vi "xy_graph_copy_format.vi"(6 "xy_scales_to_copy":i32=1, 8 "error in (no error)":errorcluster, 10 "destination":refnum<vi>, 11 "source":refnum<vi>) -> (0 "error out":errorcluster)   [LabVIEW 2015, in "lv-graph.lvlib"]
uses:
  lv-graph.lvlib
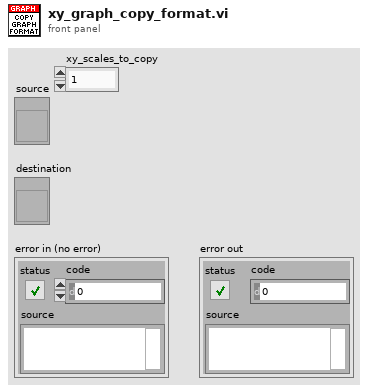
[diagram p1: front panel]
types:
  T1 = typedef "LVRangeTypeDef.ctl" = cluster{"Minimum":dbl, "Maximum":dbl, "Increment":dbl, "Minor Increment":dbl, "Start":dbl}
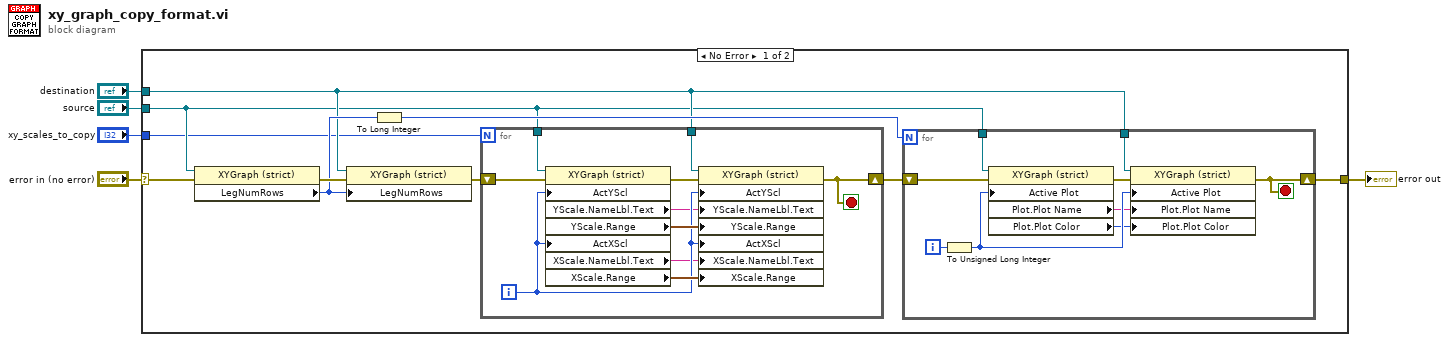
[diagram p0: block diagram]
diagram:
  n1 = case shown="No Error" "error in (no error)" {
    selector: "error in (no error)" -> [w7 w35]
    tunnel: [w12 w35] -> w5
    tunnel: "destination" -> [w9 _]
    tunnel: "source" -> [w8 _]
    tunnel: "xy_scales_to_copy" -> [w6 _]
    frame No Error {
      n2 = property class="XYGraph (strict)"(reference=w8, error in=w7) -> (error out=w15:errorcluster, "LegNumRows"=w14:u32)  [unwired: 1 out]
      n3 = property on="Property Node" class="XYGraph (strict)"(reference=w9, error in=w15, "LegNumRows"=w14) -> (error out=w11:errorcluster)  [unwired: 1 out]
      n4 = To Long Integer(number=w14) -> (32bit integer=w13:i32)
      n5 = for {
        N: w6 -> [_]
        shift-right: [w22] -> w10
        shift-left: w11 -> [w23]
        tunnel: w8 -> [w21]
        tunnel: w9 -> [w20]
        i -> [w18]
        stop <- w22 stop-if-true
        n6 = property on="Property Node" class="XYGraph (strict)"(reference=w21, error in=w23, "ActYScl"=w18, "ActXScl"=w18) -> (error out=w25:errorcluster, "YScale.NameLbl.Text"=w16:string, "YScale.Range"=w24:T1, "XScale.NameLbl.Text"=w17:string, "XScale.Range"=w19:T1)  [unwired: 1 out]
        n7 = property on="Property Node" class="XYGraph (strict)"(reference=w20, error in=w25, "ActYScl"=w18, "YScale.NameLbl.Text"=w16, "YScale.Range"=w24, "ActXScl"=w18, "XScale.NameLbl.Text"=w17, "XScale.Range"=w19) -> (error out=w22:errorcluster)  [unwired: 1 out]
      }
      n8 = for {
        N: w13 -> [_]
        shift-right: [w28] -> w12
        shift-left: w10 -> [w33]
        tunnel: w9 -> [w27]
        tunnel: w8 -> [w26]
        i -> [w32]
        stop <- w28 stop-if-true
        n9 = To Unsigned Long Integer(number=w32) -> (unsigned 32bit integer=w34:u32)
        n10 = property class="XYGraph (strict)"(reference=w26, error in=w33, "Active Plot"=w34) -> (error out=w31:errorcluster, "Plot.Plot Name"=w30:string, "Plot.Plot Color"=w29:u32)  [unwired: 1 out]
        n11 = property on="Property Node" class="XYGraph (strict)"(reference=w27, error in=w31, "Active Plot"=w34, "Plot.Plot Name"=w30, "Plot.Plot Color"=w29) -> (error out=w28:errorcluster)  [unwired: 1 out]
      }
    }
    frame Error {
    }
  }
  "error out" <- w5
